vi "Verify Permissions PDFReader.vi"(7 "File and pages":T1={"Path"=path "", "Pages"="all", "Password"=""}, 11 "error in (no error)":errorcluster) -> (8 "Allow copy?":bool, 15 "error out":errorcluster)   [LabVIEW 2019, in "Exaprom PDF.lvlib"]
doc: "Version 1.1\nDeveloped by Jean-Marc Simard\nCopyright © 2012, Exaprom Inc.\nAll rights reserved.\nLicense: BSD\n\nWith iTextSharp 4.1.6 (http://itextsharp.sourceforge.net)\nunder Mozilla Public License Version 1.1\n(http://www.mozilla.org/MPL/MPL-1.1.html)"
uses:
  Controls/Concatenate Controls/PDF file to concatenate.ctl
  C:/work/niobrara_lv/labview pdf writer fixing/DLL/itextsharp.dll
  DLL/itextsharp.dll
  Exaprom PDF.lvlib
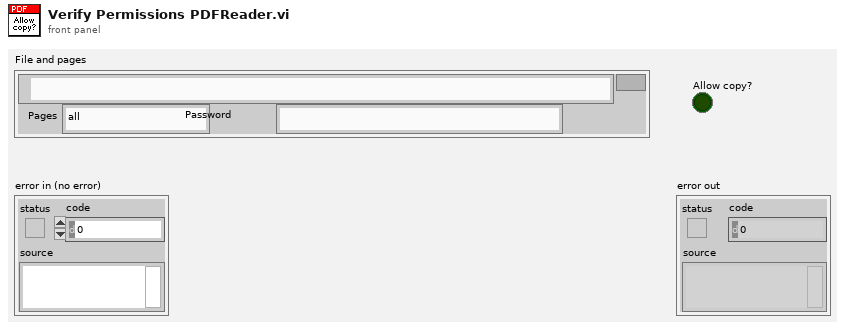
[diagram p1: front panel]
types:
  T1 = typedef "Exaprom PDF.lvlib/PDF file to concatenate.ctl" = cluster{"Path":path, "Pages":string, "Password":string}
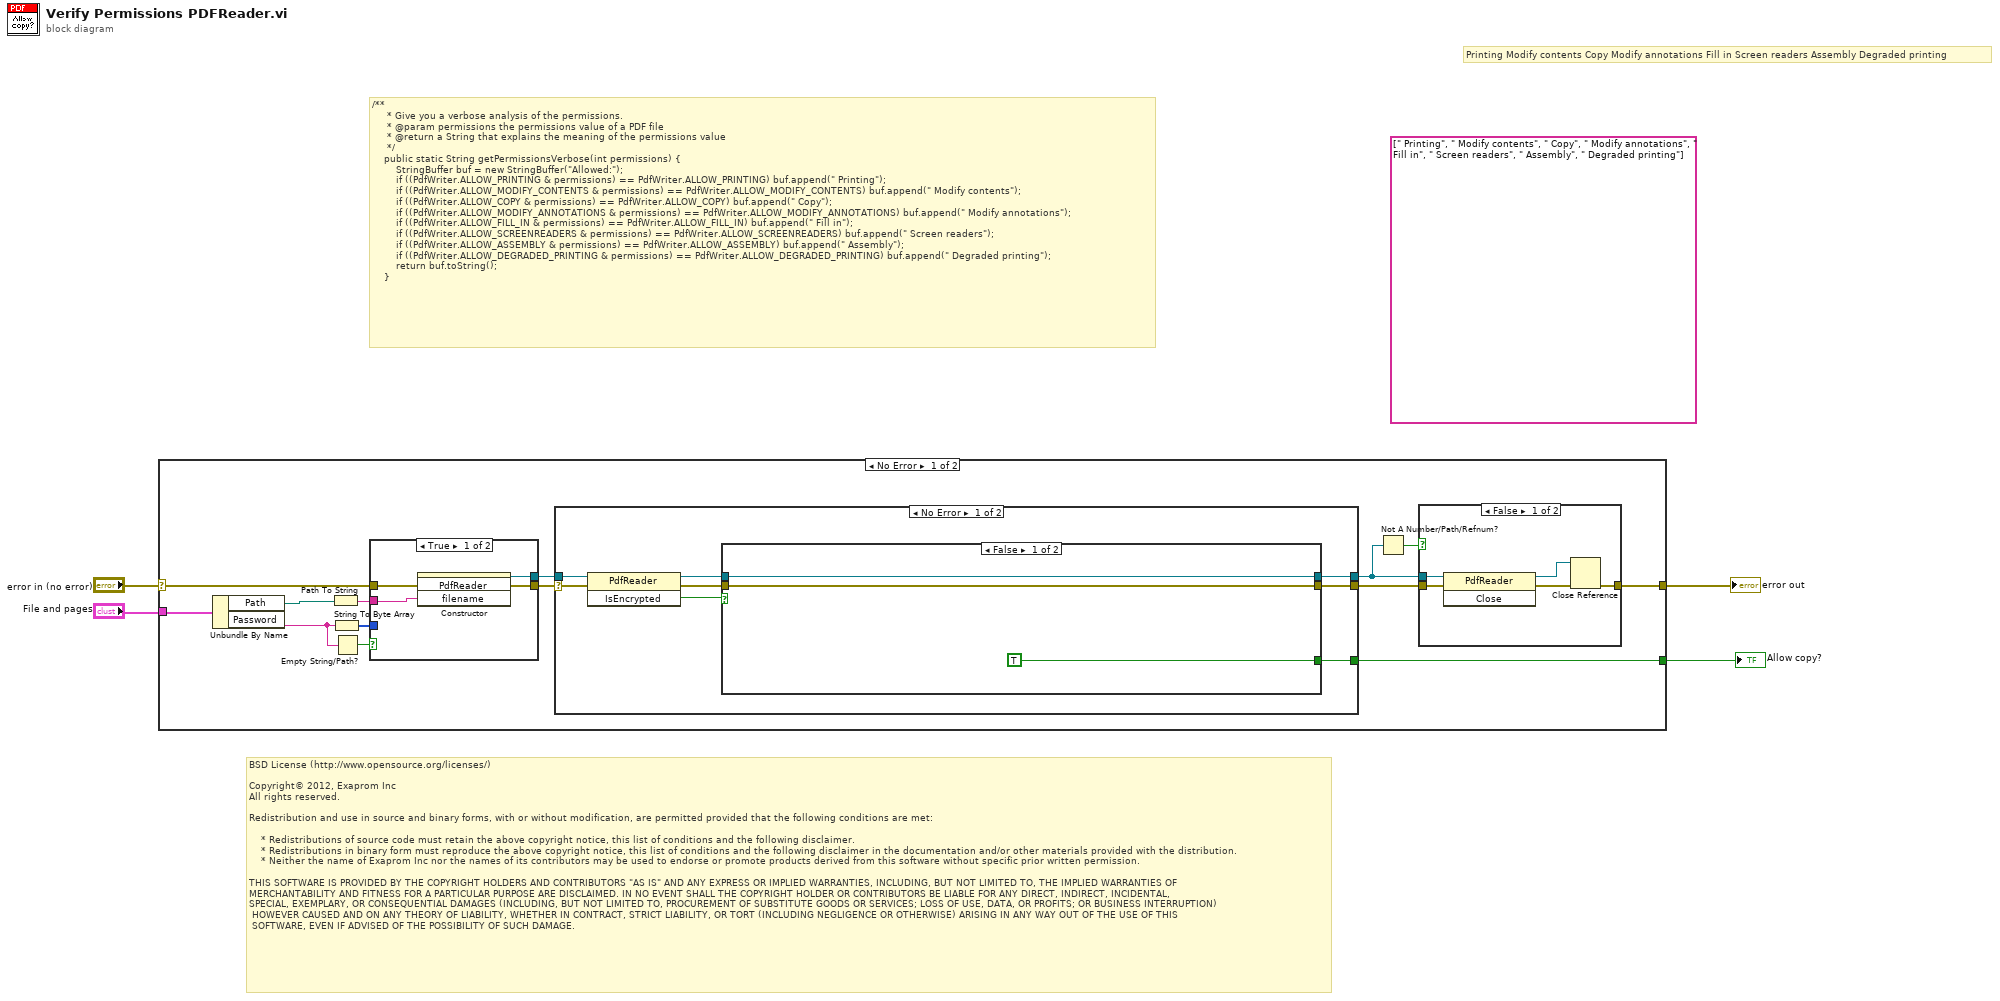
[diagram p0: block diagram]
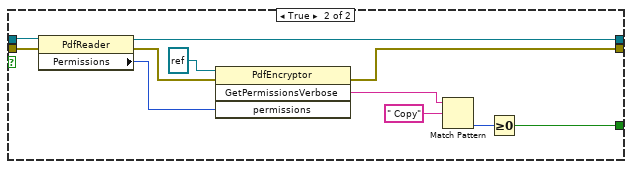
[diagram p3: hidden frame]
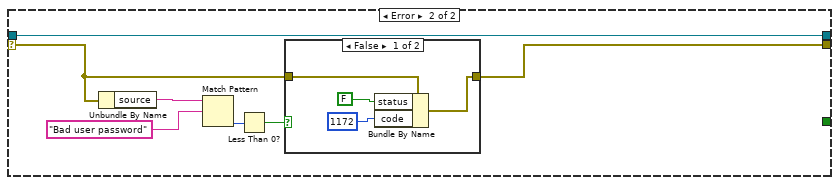
[diagram p4: hidden frame]
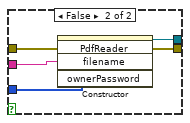
[diagram p6: hidden frame]
diagram:
  (unwired) string[] [" Printing", " Modify contents", " Copy", " Modify annotations", " Fill in", " Screen readers", " Assembly", " Degraded printing"]
  # "Printing Modify contents Copy Modify annotations Fill in Screen readers Assembly Degraded printing"
  # "/**\n     * Give you a verbose analysis of the permissions.\n     * @param permissions the permissions value of a PDF file\n     * @return a String that explains the meaning of the permissions value\n     */\n    public static String getPermissionsVerbose(int permissions) {\n        StringBuffer buf = new StringBuffer(\"Allowed:\");\n        if ((PdfWriter.ALLOW_PRINTING & permissions) == PdfWriter.ALLOW_PRINTING) buf.append(\" Printing\");\n        if ((PdfWriter.ALLOW_MODIFY_CONTENTS & permissions) == PdfWriter.ALLOW_MODIFY_CONTENTS) buf.append(\" Modify contents\");\n        if ((PdfWriter.ALLOW_COPY & permissions) == PdfWriter.ALLOW_COPY) buf.append(\" Copy\");\n        if ((PdfWriter.ALLOW_MODIFY_ANNOTATIONS & permissions) == PdfWriter.ALLOW_MODIFY_ANNOTATIONS) buf.append(\" Modify annotations\");\n        if ((PdfWriter.ALLOW_FILL_IN & permissions) == PdfWriter.ALLOW_FILL_IN) buf.append(\" Fill in\");\n        if ((PdfWriter.ALLOW_SCREENREADERS & permissions) == PdfWriter.ALLOW_SCREENREADERS) buf.append(\" Screen readers\");\n        if ((PdfWriter.ALLOW_ASSEMBLY & permissions) == PdfWriter.ALLOW_ASSEMBLY) buf.append(\" Assembly\");\n        if ((PdfWriter.ALLOW_DEGRADED_PRINTING & permissions) == PdfWriter.ALLOW_DEGRADED_PRINTING) buf.append(\" Degraded printing\");\n        return buf.toString();\n    }"
  # "BSD License (http://www.opensource.org/licenses/)\n\nCopyright© 2012, Exaprom Inc\nAll rights reserved.\n\nRedistribution and use in source and binary forms, with or without modification, are permitted provided that the following conditions are met:\n\n    * Redistributions of source code must retain the above copyright notice, this list of conditions and the following disclaimer.\n    * Redistributions in binary form must reproduce the above copyright notice, this list of conditions and the following disclaimer in the documentation and/or other materials provided with the distribution.\n    * Neither the name of Exaprom Inc nor the names of its contributors may be used to endorse or promote products derived from this software without specific prior written permission.\n\nTHIS SOFTWARE IS PROVIDED BY THE COPYRIGHT HOLDERS AND CONTRIBUTORS \"AS IS\" AND ANY EXPRESS OR IMPLIED WARRANTIES, INCLUDING, BUT NOT LIMITED TO, THE IMPLIED WARRANTIES OF \nMERCHANTABILITY AND FITNESS FOR A PARTICULAR PURPOSE ARE DISCLAIMED. IN NO EVENT SHALL THE COPYRIGHT HOLDER OR CONTRIBUTORS BE LIABLE FOR ANY DIRECT, INDIRECT, INCIDENTAL,\nSPECIAL, EXEMPLARY, OR CONSEQUENTIAL DAMAGES (INCLUDING, BUT NOT LIMITED TO, PROCUREMENT OF SUBSTITUTE GOODS OR SERVICES; LOSS OF USE, DATA, OR PROFITS; OR BUSINESS INTERRUPTION)\n HOWEVER CAUSED AND ON ANY THEORY OF LIABILITY, WHETHER IN CONTRACT, STRICT LIABILITY, OR TORT (INCLUDING NEGLIGENCE OR OTHERWISE) ARISING IN ANY WAY OUT OF THE USE OF THIS\n SOFTWARE, EVEN IF ADVISED OF THE POSSIBILITY OF SUCH DAMAGE."
  n1 = case shown="No Error" "error in (no error)" {
    selector: "error in (no error)" -> [w7 w68]
    tunnel: [w16 w68] -> w4
    tunnel: "File and pages" -> [w18 _]
    tunnel: [w8 _] -> w1
    frame No Error {
      n2 = Unbundle By Name(w18) -> ("Path"=w17:path, "Password"=w12:string)
      n3 = Path To String(path=w17) -> (string=w13:string)
      n4 = String To Byte Array(string=w12) -> (unsigned byte array=w10:u8[])
      n5 = Empty String/Path?(string/path=w12) -> (empty?=w11:bool)
      n6 = case shown="True" w11 {
        tunnel: w7 -> [w62 w67]
        tunnel: w13 -> [w61 w66]
        tunnel: [w60 w65] -> w15
        tunnel: [w59 w64] -> w9
        tunnel: w10 -> [_ w63]
        frame True {
          n7 = constructor class="PdfReader"(error in=w62, "filename"=w61) -> (reference out=w60:refnum<k24>, error out=w59:errorcluster)  [unwired: 2 in, 2 out]
        }
        frame False {
          n8 = constructor class="PdfReader"(error in=w67, "filename"=w66, "ownerPassword"=w63) -> (reference out=w65:refnum<k24>, error out=w64:errorcluster)  [unwired: 2 in, 3 out]
        }
      }
      n9 = case shown="No Error" w9 {
        selector: w9 -> [w26 w48]
        tunnel: w15 -> [w32 w53]
        tunnel: [w29 w47] -> w14
        tunnel: [w28 w53] -> w5
        tunnel: [w25 _] -> w8
        frame No Error {
          n10 = invoke class="PdfReader" method="IsEncrypted"(reference=w32, error in=w26) -> (reference out=w31:refnum<k24>, error out=w30:errorcluster, "IsEncrypted"=w27:bool)  [unwired: 1 in]
          n11 = case shown="False" w27 {
            tunnel: w31 -> [w35 w44]
            tunnel: w30 -> [w34 w45]
            tunnel: [w34 w40] -> w29
            tunnel: [w35 w46] -> w28
            tunnel: [TRUE w36] -> w25
            frame False {
            }
            frame True {
              n12 = property class="PdfReader"(reference=w44, error in=w45) -> (reference out=w46:refnum<k24>, error out=w41:errorcluster, "Permissions"=w42:i32)
              n13 = invoke class="PdfEncryptor" method="GetPermissionsVerbose"(reference=refnum<k24> refnum ("new reference"), error in=w41, "permissions"=w42) -> (error out=w40:errorcluster, "GetPermissionsVerbose"=w39:string)  [unwired: 1 in, 2 out]
              n14 = Match Pattern(string=w39, regular expression=" Copy") -> (offset past match=w37:i32)  [unwired: 1 in, 3 out]
              n15 = Greater Or Equal To 0?(x=w37) -> (x >= 0?=w36:bool)
            }
          }
        }
        frame Error {
          n16 = Unbundle By Name(w48) -> ("source"=w52:string)
          n17 = Match Pattern(string=w52, regular expression="Bad user password") -> (offset past match=w50:i32)  [unwired: 1 in, 3 out]
          n18 = Less Than 0?(x=w50) -> (x < 0?=w49:bool)
          n19 = case shown="False" w49 {
            tunnel: w48 -> [w57 w58]
            tunnel: [w54 w58] -> w47
            frame False {
              n20 = Bundle By Name(cluster=w57, "status"=FALSE, "code"=1172) -> (w54:errorcluster)
            }
            frame True {
            }
          }
        }
      }
      n21 = Not A Number/Path/Refnum?(number/path/refnum=w5) -> (NaN/Path/Refnum?=w6:bool)
      n22 = case shown="False" w6 {
        tunnel: [w23 w24] -> w16
        tunnel: w14 -> [w20 w24]
        tunnel: w5 -> [w19 _]
        frame False {
          n23 = invoke class="PdfReader" method="Close"(reference=w19, error in=w20) -> (reference out=w21:refnum<k24>, error out=w22:errorcluster)  [unwired: 1 in, 1 out]
          n24 = Close Reference(reference=w21, error in (no error)=w22) -> (error out=w23:errorcluster)
        }
        frame True {
        }
      }
    }
    frame Error {
    }
  }
  "error out" <- w4
  "Allow copy?" <- w1
